vi "sc5511a_soft_front_panel.vi"() -> ()   [LabVIEW 2010]
panel:
  out "message":string="List/Sweep Mode Disabled"
  out "On":bool
  in  "stop":bool
  in  "Tab Control":T1(tab)
  in  "Phase":sgl min=-720 max=720 step=0.1 format="%.1f"
  in  "Spur Suppression":u8(ring) items=["Enabled", "Disabled"]
  in  "AutoLevel":u8(ring) items=["Enable", "Disable"]
  in  "Loop Gain":u8(ring) items=["Normal", "Low"]
  in  "Ref. Out Freq":u8(ring) items=["10 MHz", "100 MHz"]
  in  "Ref. Clock Source":u8(ring) items=["Internal 10 MHz", "Lock to External"]
  in  "RF1 Standby":bool
  in  "Lock Mode":u8(ring) items=["Harmonic Lock", "Frac-N Lock"]
  in  "ALC MODE":u8(ring) items=["Closed", "Opened"]
  in  "Power":sgl=30.0 min=-40 max=30 format="%.2f"
  in  "Interval (s)":u16=5
  in  "GetStatus":bool
  in  "Trigger":bool
  out "Device Status":T2={"Synth Mode"=1, "RF Out"=0, "Auto Level"=0, "ALC Mode"=1, "Standby"=1, "Rf RF Mode"=0, "List Mode State"=0, "RF2 Standby"=0, "Ref Lock Enable"=1, "Ext Ref Detected"=1, "Ref out mode"=1, "Main PLL"=1, "Crs PLL"=1, "Fine PLL"=1, "device accessed"=0, "Over Temp"=0, "MainLED"=FALSE, "CrsLED"=FALSE, "FineLED"=FALSE} {"Over Temp" items=["Normal", "Over Temp"]; "Ref out mode" items=["10 MHz", "100 MHz"]; "device accessed" items=["NO", "YES"]; "RF2 Standby" items=["Disabled", "Enabled"]; "Standby" items=["Disable", "Enabled"]; "Auto Level" items=["Enable", "Disable"]; "Ext Ref Detected" items=["Not Detected", "Detected"]; "Ref Lock Enable" items=["Disabled", "Enabled"]; "RF Out" items=["Disabled", "Enabled"]; "ALC Mode" items=["Closed", "Opened"]; "Rf RF Mode" items=["Single Tone", "List/Sweep"]; "Synth Mode" items=["Harmonic", "FracN"]; "List Mode State" items=["Not Triggered", "Triggered"]; "Main PLL" items=["NOT Locked", "Locked"]; "Crs PLL" items=["NOT Locked", "Locked"]; "Fine PLL" items=["NOT Locked", "Locked"]}
  in  "RF Frequency":dbl=2005000000.0 min=80000000.0 max=21000000000.0 step=1.0 format="%.9p"
  in  "RF Mode":u8(ring) items=["Single Tone", "List/Sweep"]
  in  "RF Enable":bool
  in  "RF2 Freq":sgl=6000.0 min=25 max=6000 step=25
  in  "RF2 Standby":bool
  in  "Set As Default":bool
  in  "Dwell Period (ms)":dbl=10.0 min=0.0 step=0.5 format="%.1f"
  in  "Sweep/List Cycles":u32
  in  "Sweep Freq Parameter":T3={"Start Frequency"=10040000000, "Stop Frequency"=10050000000, "Step Frequency"=100000} {"Step Frequency" max=6500000000 format="%.9p"; "Stop Frequency" max=21000000000 format="%.9p"; "Start Frequency" format="%.9p"}
  in  "List Mode Config":T4={"Sweep / List"=1, "Direction"=0, "Shape"=1, "Trigger Source"=1, "HW Trigger Mode"=0, "Return to Start"=0, "Trigger Out State"=1, "Trigger Out Behavior"=0} {"Trigger Out Behavior" items=["Trigger On Step", "Trigger On Cycle"]; "Trigger Out State" items=["Trigger Out Disable", "Trigger Out Enable"]; "Return to Start" items=["Stop at End", "Return to Start"]; "HW Trigger Mode" items=["Start/Stop", "Step"]; "Trigger Source" items=["Software", "Hardware"]; "Shape" items=["Sawtooth", "Triangle"]; "Direction" items=["Low to High", "High to Low"]; "Sweep / List" items=["List", "Sweep (start/stop/step)"]}
  in  "Load Config":bool
  in  "Save Buffer to EEPROM":bool
  in  "Read EEPROM to Buffer":bool
  in  "Download to Buffer":bool
  in  "Read From File":bool
  in  "Frequency List (2048 max)":u64[](array[numeric]) format="%.9p"
  out "message 2":string
  out "List Points":u32
  in  "SelfCal":bool
  out "Temperature":sgl=40.0 min=-30 max=120 format="%.1f"
  out "Device Info":T5={"Product SN"=268435879, "Hardware Rev"=2.0, "Firmware Rev"=2.0, "Manuf Date"={"Year"=14, "Month"=9, "Day"=10, "Hour"=10}} {"Firmware Rev" format="%.2g"; "Hardware Rev" format="%.2g"; "Product SN" format="%.0x"}
  out "error out":errorcluster
  # "(Deg)"
  # "MHz"
  # "Program will stop and the device will \nreinitialize after self calibration"
  # "DegC"
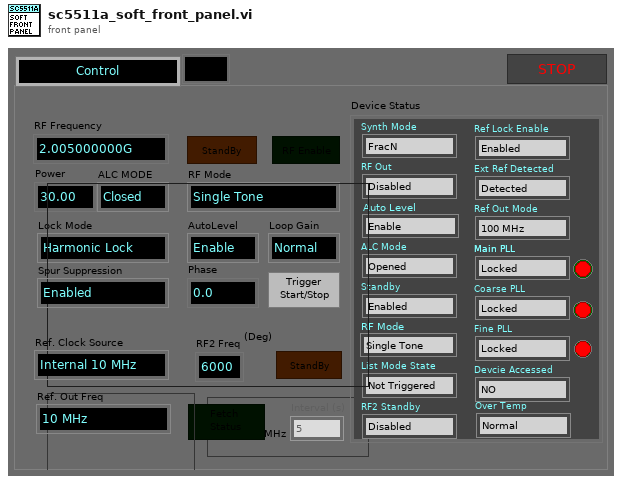
[diagram p1: front panel]
types:
  T1 = enum32{"Control", "Config Sweep/List", "List Entry", "Device Info"}
  T2 = cluster{"Synth Mode":u16, "RF Out":u16, "Auto Level":u16, "ALC Mode":u16, "Standby":u16, "Rf RF Mode":u16, "List Mode State":u16, "RF2 Standby":u16, "Ref Lock Enable":u16, "Ext Ref Detected":u16, "Ref out mode":u16, "Main PLL":u8, "Crs PLL":u8, "Fine PLL":u8, "device accessed":u16, "Over Temp":u16, "MainLED":bool, "CrsLED":bool, "FineLED":bool}
  T3 = cluster{"Start Frequency":u64, "Stop Frequency":u64, "Step Frequency":u64}
  T4 = cluster{"Sweep / List":u8, "Direction":u8, "Shape":u8, "Trigger Source":u8, "HW Trigger Mode":u8, "Return to Start":u8, "Trigger Out State":u8, "Trigger Out Behavior":u8}
  T5 = cluster{"Product SN":u32, "Hardware Rev":sgl, "Firmware Rev":sgl, "Manuf Date":cluster{"Year":u8, "Month":u8, "Day":u8, "Hour":u8}}
  T6 = cluster{"Product SN":u32, "Hardware Rev":sgl, "Firmware Rev":sgl, "Manuf Date":cluster{"Year":u32, "Month":u32, "Day":u32, "hour":u32}}
  T7 = enum32{"Control", "Config Sweep/List", "List Entry"}
  T8 = enum8{"Enabled", "Disabled", "Disabled and Grayed Out"}
  T9 = cluster{"Synth Mode":u16, "RF Out":u16, "Auto Power":u16, "ALC Mode":u16, "Standby":u16, "Rf RF Mode":u16, "List Mode State":u16, "RF2 Standby":u16, "Ref Lock Enable":u16, "Ext Ref Detected":u16, "Ref out mode":u16, "Main PLL":u8, "Crs PLL":u8, "Fine PLL":u8, "device accessed":u16, "Over Temp":u16, "MainLED":bool, "CrsLED":bool, "FineLED":bool}
  T10 = cluster{"Product SN":u32, "Hardware Rev":sgl, "Firmware Rev":sgl, "Manufacture Date":cluster{"Year":u8, "Month":u8, "Day":u8, "hour":u8}}
  T11 = cluster{"List Mode Config":cluster{"List/SSS":u8, "Direction":u8, "Shape":u8, "Trigger Source":u8, "HW Trigger Mode":u8, "Return to Start":u8, "Trigger Out State":u8, "Trigger Out Behavior":u8}, "Operate Status":cluster{"Lock Mode":u8, "Loop Gain":u8, "Device Accessed":u8, "RF2 Standby":u8, "RF1 Standby":u8, "AutoPwrLevel":u8, "AlcMode":u8, "RFOutState":u8, "Ref Lock Enable":u8, "ExtRefDetected":u8, "RefOutSelect":u8, "ListRuning":u8, "RF Mode":u8, "OverTempStatus":u8, "Harmonic SS":u8}, "PLL Status":cluster{"Sum PLL":u8, "Crs PLL":u8, "Fine PLL":u8, "Crs Ref PLL":u8, "Crs assist PLL":u8, "Ref Clk PLL":u8, "Clk 10 PLL":u8, "Lo2 PLL":u8}}
  T12 = cluster{"RF1 Freq":u64, "Sweep Start Freq":u64, "Sweep Stop Freq":u64, "Sweep Step Freq":u64, "Sweep dwell time (.5ms)":u32, "Sweep Cycles":u32, "List Buffer Points":u32, "RF1 Level (dBm)":sgl, "RF2 freq":u16}
  T13 = cluster{"List/SSS":u8, "Direction":u8, "Shape":u8, "Trigger Source":u8, "HW Trigger Mode":u8, "Return to Start":u8, "Trigger Out State":u8, "Trigger Out Behavior":u8}
  T14 = cluster{"Sweep Start Freq":u64, "Sweep Stop Freq":u64, "Sweep Step Freq":u64}
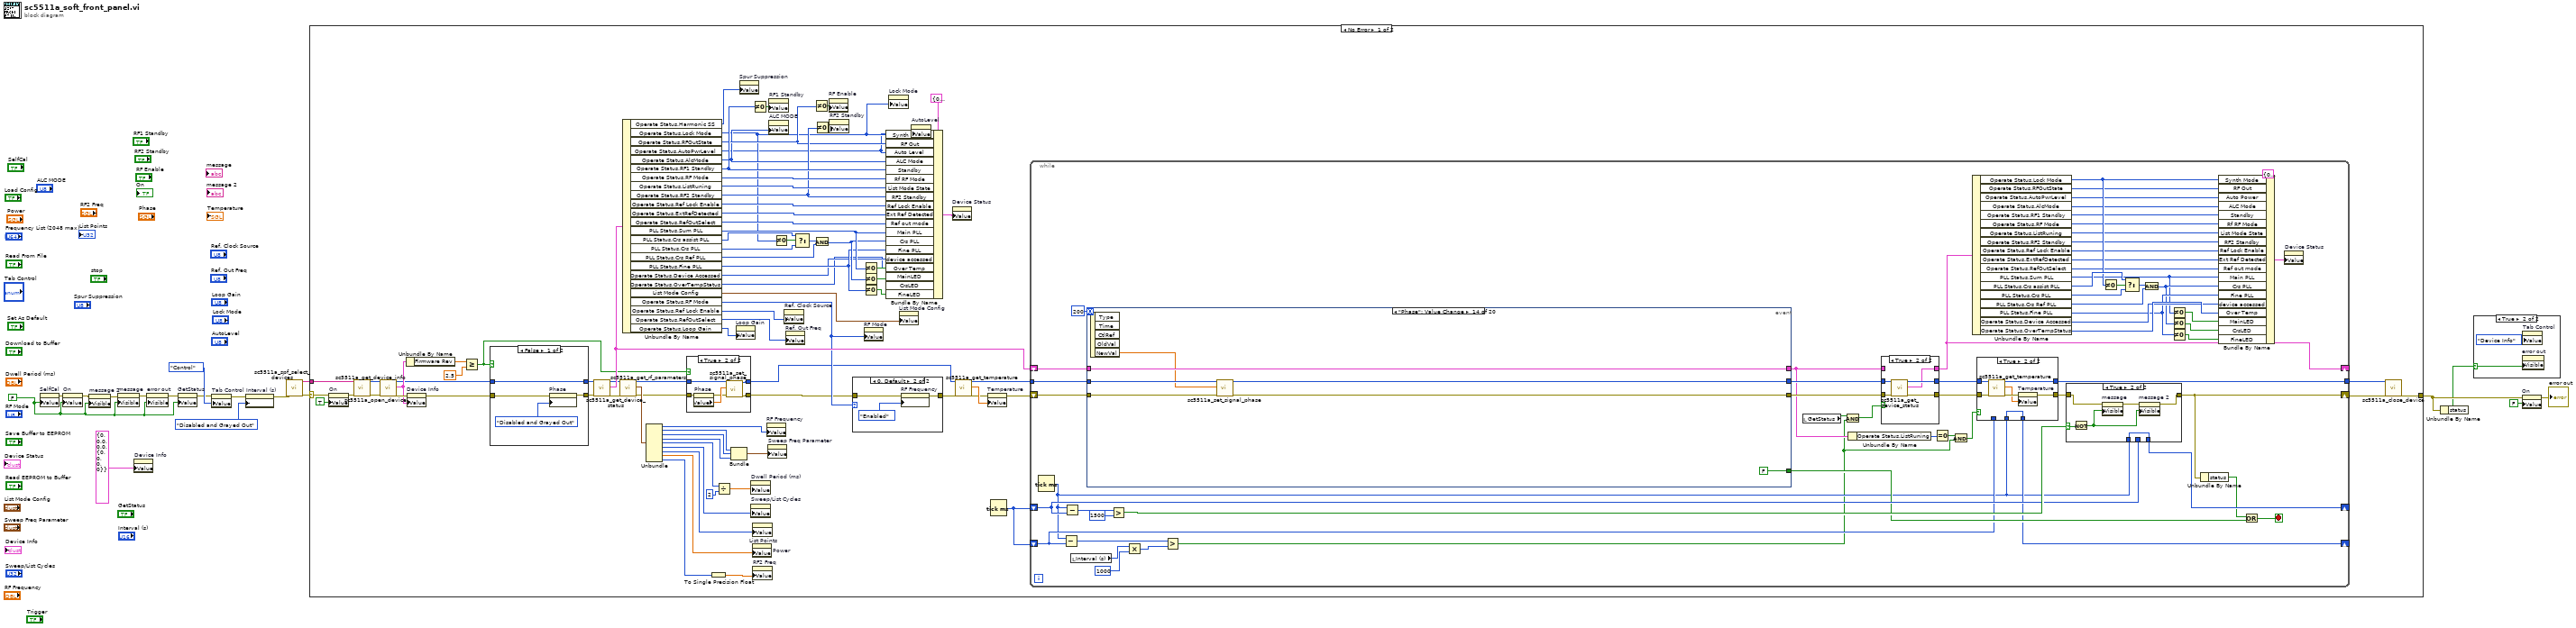
[diagram p0: block diagram]
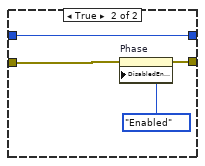
[diagram p4: hidden frame]
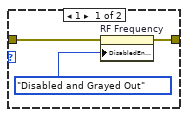
[diagram p5: hidden frame]
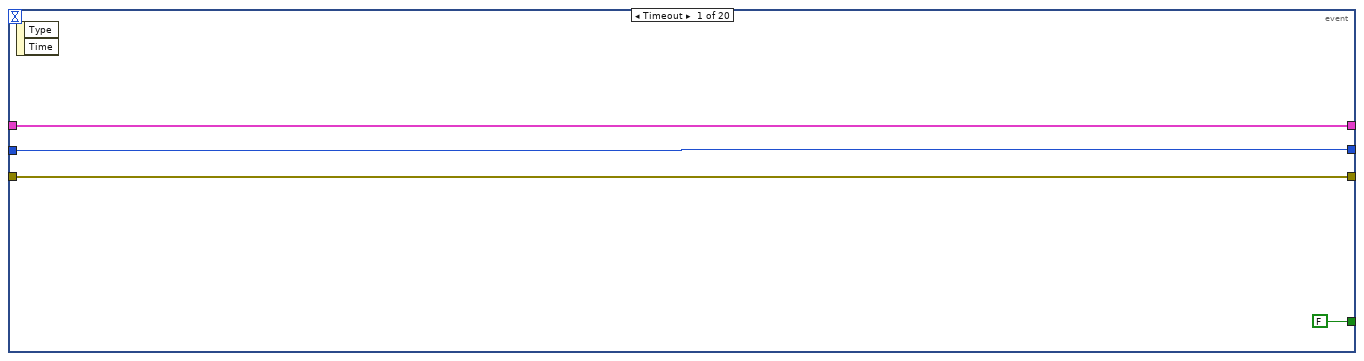
[diagram p9: hidden frame]
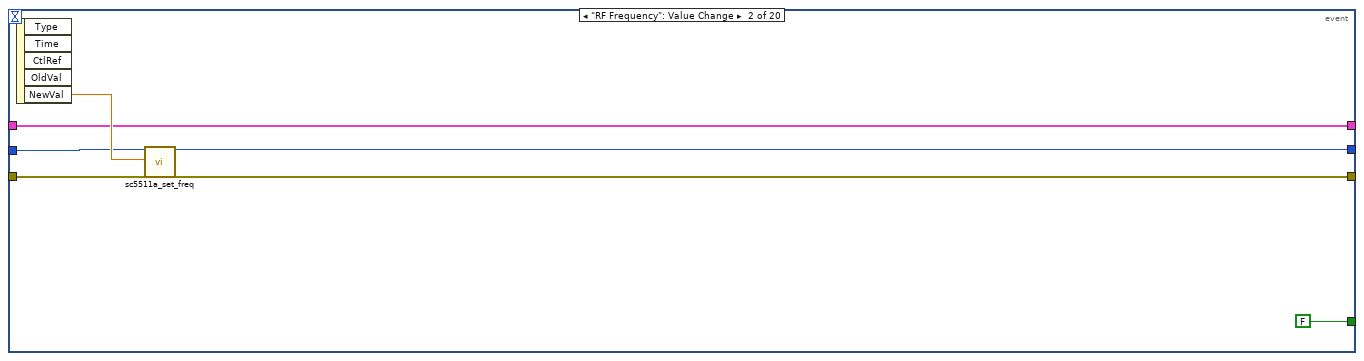
[diagram p10: hidden frame]
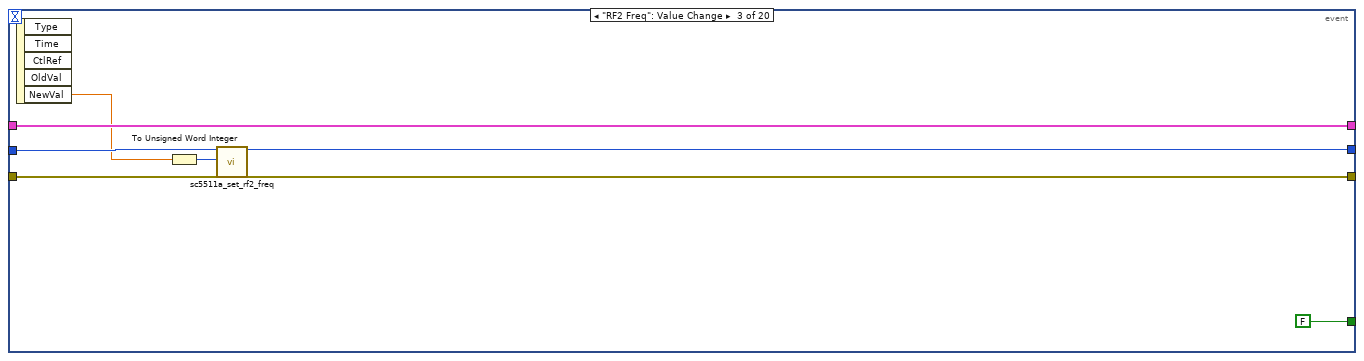
[diagram p11: hidden frame]
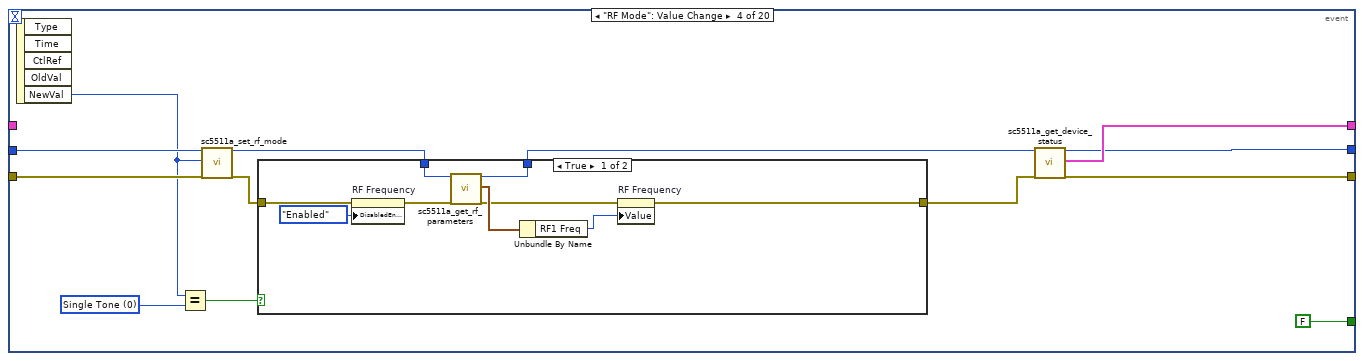
[diagram p12: hidden frame]
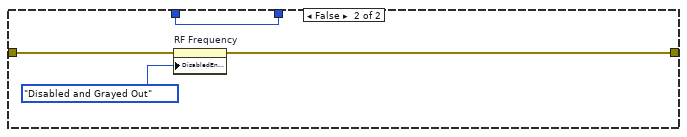
[diagram p13: hidden frame]
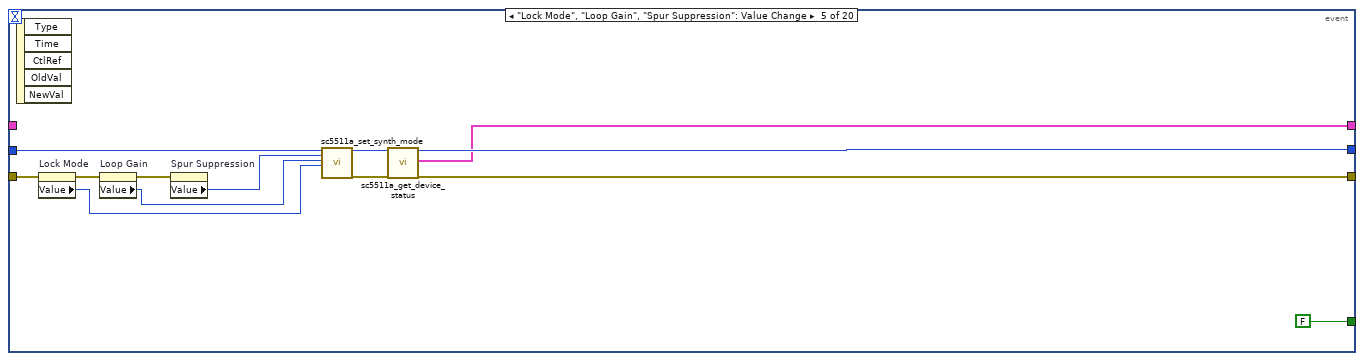
[diagram p14: hidden frame]
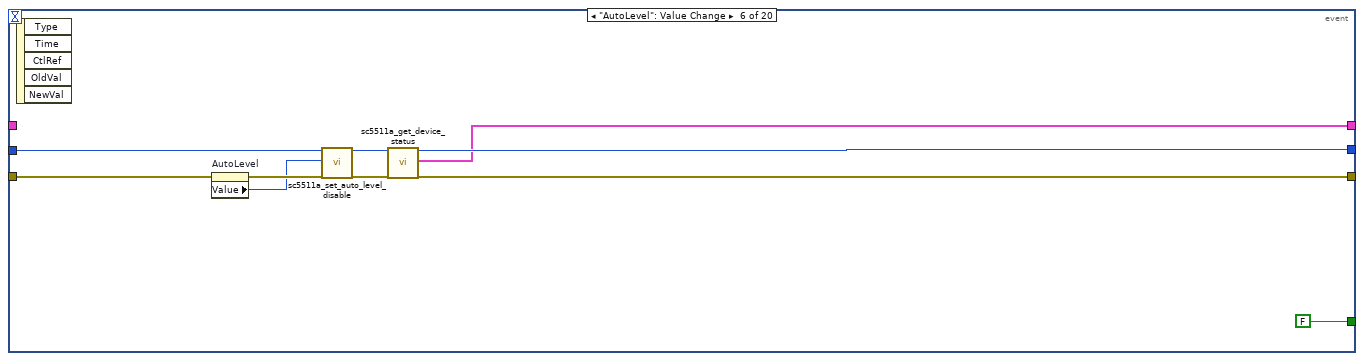
[diagram p15: hidden frame]
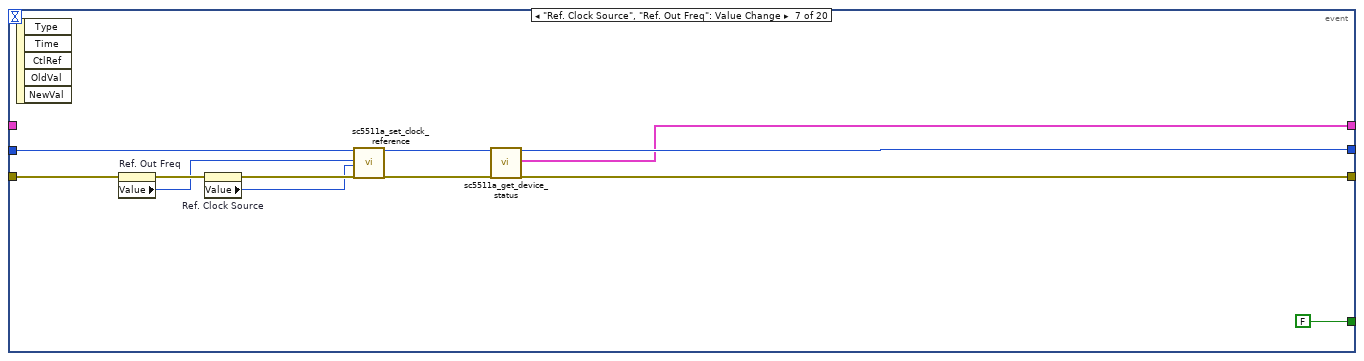
[diagram p16: hidden frame]
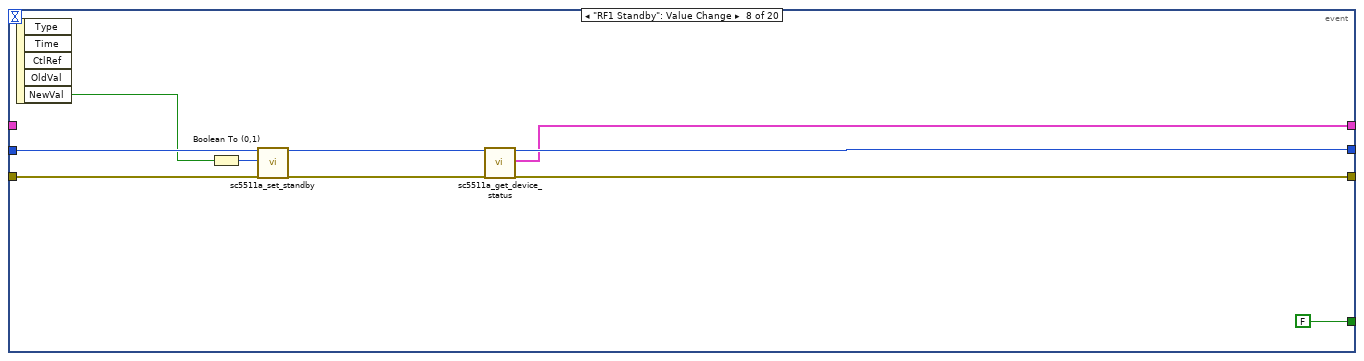
[diagram p17: hidden frame]
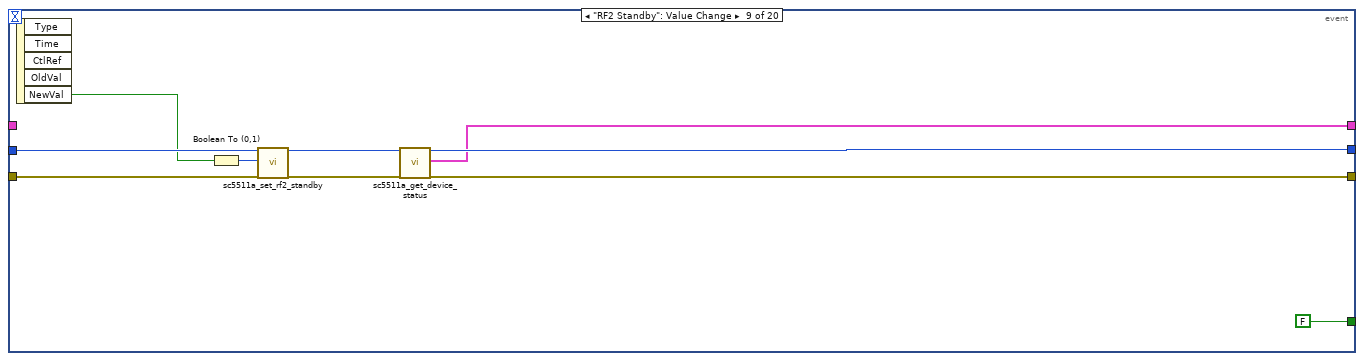
[diagram p18: hidden frame]
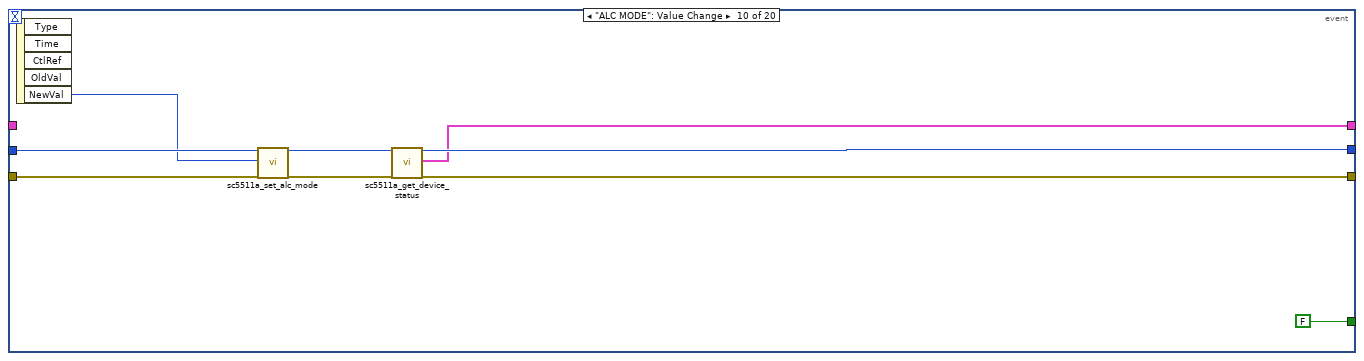
[diagram p19: hidden frame]
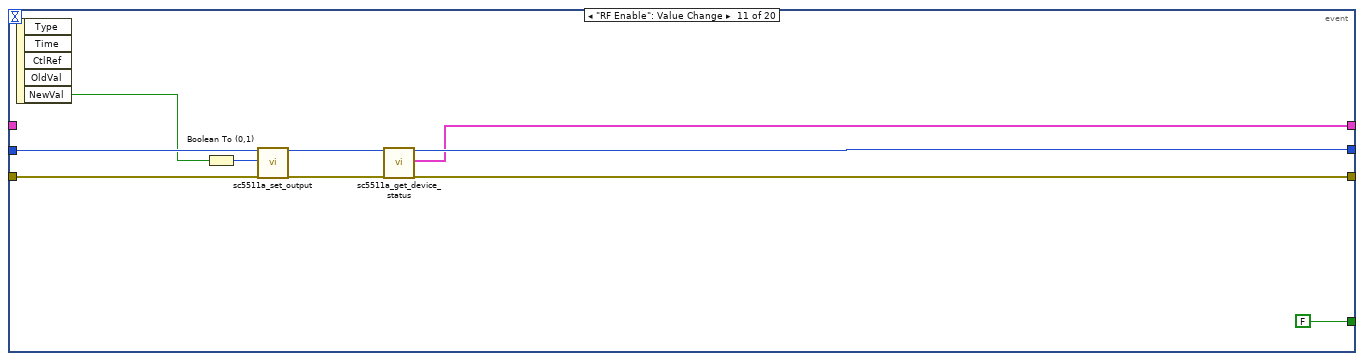
[diagram p20: hidden frame]
diagram:
  w1 = FALSE ("Visible")
  n1 = property on="SelfCal" class="Bool (strict)"("Value"=w1) -> (error out=w2:errorcluster)  [unwired: 2 in, 1 out]
  n2 = property on="On" class="Bool (strict)"(error in=w2, "Value"=w1) -> (error out=w4:errorcluster)  [unwired: 1 in, 1 out]
  n3 = property on="message 2" class="Str"(error in=w4, "Visible"=w1) -> (error out=w18:errorcluster)  [unwired: 1 in, 1 out]
  n4 = property on="message" class="Str"(error in=w18, "Visible"=w1) -> (error out=w17:errorcluster)  [unwired: 1 in, 1 out]
  n5 = property on="Device Info" class="Clust (strict)"("Value"=T6 {"Product SN"=0, "Hardware Rev"=0.0, "Firmware Rev"=0.0, "Manuf Date"={"Year"=0, "Month"=0, "Day"=0, "hour"=0}} ("Device Info")) -> ()  [unwired: 2 in, 2 out]
  n6 = property on="error out" class="Clust (strict)"(error in=w17, "Visible"=w1) -> (error out=w15:errorcluster)  [unwired: 1 in, 1 out]
  n7 = property on="GetStatus" class="Bool (strict)"(error in=w15, "Value"=w1) -> (error out=w10:errorcluster)  [unwired: 1 in, 1 out]
  n8 = property on="Tab Control" class="TabCtl (strict)"(error in=w10, "Value"=T7."Control" ("Tab Control")) -> (error out=w11:errorcluster)  [unwired: 1 in, 1 out]
  n9 = property on="Interval (s)" class="DigNum (strict)"(error in=w11, "DisabledEnum"=T8."Disabled and Grayed Out" ("Disabled")) -> (error out=w14:errorcluster)  [unwired: 1 in, 1 out]
  n10 = call "sc5511a_spf_select_devices.vi"("error in (no error)"=w14) -> ("Selected Resource"=w8:string, "error out"=w16:errorcluster)  [unwired: 17 in]
  n11 = case shown="No Error" w16 {
    selector: w16 -> [w84 w578]
    tunnel: [w96 w578] -> w7
    tunnel: w8 -> [w83 _]
    frame No Error {
      n12 = property on="On" class="Bool (strict)"(error in=w84, "Value"=TRUE ("Visible")) -> (error out=w85:errorcluster)  [unwired: 1 in, 1 out]
      n13 = call "sc5511a_open_device.vi"("Device SN String"=w83, "error in (no error)"=w85) -> ("deviceHandle"=w87:u32, "error out"=w88:errorcluster)  [unwired: 16 in]
      n14 = call "sc5511a_get_device_info.vi"("deviceHandle"=w87, "error in"=w88) -> ("deviceHandle"=w22:u32, "Device Info"=w27:T10, "error out"=w93:errorcluster)  [unwired: 15 in]
      n15 = Unbundle By Name(w27) -> ("Firmware Rev"=w26:sgl)
      n16 = property on="Device Info" class="Clust (strict)"(error in=w93, "Value"=w27) -> (error out=w23:errorcluster)  [unwired: 1 in, 1 out]
      n17 = Greater Or Equal?(x=w26, y=sgl 2.5) -> (x >= y?=w19:bool)
      n18 = case shown="False" w19 {
        tunnel: [w108 w113] -> w24
        tunnel: w23 -> [w109 w112]
        tunnel: w22 -> [w110 w114]
        tunnel: [w110 w114] -> w21
        frame False {
          n19 = property on="Phase" class="DigNum (strict)"(error in=w109, "DisabledEnum"=T8."Disabled and Grayed Out" ("Disabled")) -> (error out=w108:errorcluster)  [unwired: 1 in, 1 out]
        }
        frame True {
          n20 = property on="Phase" class="DigNum (strict)"(error in=w112, "DisabledEnum"=T8."Enabled" ("Disabled")) -> (error out=w113:errorcluster)  [unwired: 1 in, 1 out]
        }
      }
      n21 = call "sc5511a_get_device_status.vi"("deviceHandle"=w21, "error in"=w24) -> ("deviceHandle"=w80:u32, "Device Status"=w94:T11, "error out"=w81:errorcluster)  [unwired: 15 in]
      n22 = call "sc5511a_get_rf_parameters.vi"("deviceHandle"=w80, "error in"=w81) -> ("deviceHandle"=w29:u32, "RF Params"=w79:T12, "error out"=w20:errorcluster)  [unwired: 15 in]
      n23 = Unbundle By Name(w94) -> ("Operate Status.Harmonic SS"=w31:u8, "Operate Status.Lock Mode"=w35:u8, "Operate Status.RFOutState"=w43:u8, "Operate Status.AutoPwrLevel"=w32:u8, "Operate Status.AlcMode"=w42:u8, "Operate Status.RF1 Standby"=w48:u8, "Operate Status.RF Mode"=w65:u8, "Operate Status.ListRuning"=w64:u8, "Operate Status.RF2 Standby"=w44:u8, "Operate Status.Ref Lock Enable"=w63:u8, "Operate Status.ExtRefDetected"=w62:u8, "Operate Status.RefOutSelect"=w61:u8, "PLL Status.Sum PLL"=w60:u8, "PLL Status.Crs assist PLL"=w56:u8, "PLL Status.Crs PLL"=w55:u8, "PLL Status.Crs Ref PLL"=w57:u8, "PLL Status.Fine PLL"=w53:u8, "Operate Status.Device Accessed"=w52:u8, "Operate Status.OverTempStatus"=w51:u8, "List Mode Config"=w95:T13, "Operate Status.RF Mode"=w86:u8, "Operate Status.Ref Lock Enable"=w50:u8, "Operate Status.RefOutSelect"=w49:u8, "Operate Status.Loop Gain"=w36:u8)
      n24 = Unbundle(w79) -> ("RF1 Freq"=w78:u64, "Sweep Start Freq"=w76:u64, "Sweep Stop Freq"=w75:u64, "Sweep Step Freq"=w74:u64, "Sweep dwell time (.5ms)"=w71:u32, "Sweep Cycles"=w73:u32, "List Buffer Points"=w69:u32, "RF1 Level (dBm)"=w68:sgl, "RF2 freq"=w66:u16)
      n25 = case shown="True" w19 {
        tunnel: [w99 w106] -> w30
        tunnel: w29 -> [w100 w105]
        tunnel: [w100 w104] -> w28
        tunnel: w20 -> [w99 w102]
        frame False {
        }
        frame True {
          n26 = property on="Phase" class="DigNum (strict)"(error in=w102) -> (error out=w101:errorcluster, "Value"=w103:sgl)  [unwired: 1 in, 1 out]
          n27 = call "sc5511a_set_signal_phase.vi"("deviceHandle"=w105, "Phase (deg)"=w103, "error in"=w101) -> ("deviceHandle"=w104:u32, "error out"=w106:errorcluster)  [unwired: 15 in]
        }
      }
      n28 = To Single Precision Float(number=w66) -> (single precision float=w67:sgl)
      n29 = Divide(x=w71, y=u32 2) -> (x/y=w72:dbl)
      n30 = Bundle("Sweep Start Freq"=w76, "Sweep Stop Freq"=w75, "Sweep Step Freq"=w74) -> (w77:T14)  [unwired: 1 in]
      n31 = property on="Loop Gain" class="Ring (strict)"("Value"=w36) -> ()  [unwired: 2 in, 2 out]
      n32 = property on="Spur Suppression" class="Ring (strict)"("Value"=w31) -> ()  [unwired: 2 in, 2 out]
      n33 = property on="Dwell Period (ms)" class="DigNum (strict)"("Value"=w72) -> ()  [unwired: 2 in, 2 out]
      n34 = property on="Sweep/List Cycles" class="DigNum (strict)"("Value"=w73) -> ()  [unwired: 2 in, 2 out]
      n35 = Not Equal To 0?(x=w48) -> (x != 0?=w47:bool)
      n36 = property on="Power" class="DigNum (strict)"("Value"=w68) -> ()  [unwired: 2 in, 2 out]
      n37 = property on="List Points" class="DigNum (strict)"("Value"=w69) -> ()  [unwired: 2 in, 2 out]
      n38 = property on="RF2 Freq" class="DigNum (strict)"("Value"=w67) -> ()  [unwired: 2 in, 2 out]
      n39 = property on="RF Frequency" class="DigNum (strict)"("Value"=w78) -> ()  [unwired: 2 in, 2 out]
      n40 = property on="Sweep Freq Parameter" class="Clust (strict)"("Value"=w77) -> ()  [unwired: 2 in, 2 out]
      n41 = property on="RF1 Standby" class="Bool (strict)"("Value"=w47) -> ()  [unwired: 2 in, 2 out]
      n42 = property on="ALC MODE" class="Ring (strict)"("Value"=w42) -> ()  [unwired: 2 in, 2 out]
      n43 = Not Equal To 0?(x=w35) -> (x != 0?=w59:bool)
      n44 = property on="Ref. Clock Source" class="Ring (strict)"("Value"=w50) -> ()  [unwired: 2 in, 2 out]
      n45 = property on="Ref. Out Freq" class="Ring (strict)"("Value"=w49) -> ()  [unwired: 2 in, 2 out]
      n46 = Select(t=w56, s=w59, f=w55) -> (s? t:f=w58:u8)
      n47 = Not Equal To 0?(x=w43) -> (x != 0?=w46:bool)
      n48 = Not Equal To 0?(x=w44) -> (x != 0?=w45:bool)
      n49 = And(x=w58, y=w57) -> (x .and. y?=w54:u8)
      n50 = property on="RF Enable" class="Bool (strict)"("Value"=w46) -> ()  [unwired: 2 in, 2 out]
      n51 = property on="RF2 Standby" class="Bool (strict)"("Value"=w45) -> ()  [unwired: 2 in, 2 out]
      n52 = case shown="0, Default" w86 {
        tunnel: w30 -> [w116 w119]
        tunnel: [w115 w118] -> w40
        frame 1 {
          n53 = property on="RF Frequency" class="DigNum (strict)"(error in=w116, "DisabledEnum"=T8."Disabled and Grayed Out" ("Disabled")) -> (error out=w115:errorcluster)  [unwired: 1 in, 1 out]
        }
        frame 0, Default {
          n54 = property on="RF Frequency" class="DigNum (strict)"(error in=w119, "DisabledEnum"=T8."Enabled" ("Disabled")) -> (error out=w118:errorcluster)  [unwired: 1 in, 1 out]
        }
      }
      n55 = Not Equal To 0?(x=w60) -> (x != 0?=w91:bool)
      n56 = Not Equal To 0?(x=w54) -> (x != 0?=w90:bool)
      n57 = Not Equal To 0?(x=w53) -> (x != 0?=w89:bool)
      n58 = property on="RF Mode" class="Ring (strict)"("Value"=w86) -> ()  [unwired: 2 in, 2 out]
      n59 = Bundle By Name(cluster=T2 {"Synth Mode"=0, "RF Out"=1, "Auto Level"=1, "ALC Mode"=0, "Standby"=0, "Rf RF Mode"=0, "List Mode State"=0, "RF2 Standby"=1, "Ref Lock Enable"=0, "Ext Ref Detected"=0, "Ref out mode"=0, "Main PLL"=1, "Crs PLL"=1, "Fine PLL"=1, "device accessed"=1, "Over Temp"=0, "MainLED"=TRUE, "CrsLED"=TRUE, "FineLED"=TRUE} ("Device Status"), "Synth Mode"=w35, "RF Out"=w43, "Auto Level"=w32, "ALC Mode"=w42, "Standby"=w48, "Rf RF Mode"=w65, "List Mode State"=w64, "RF2 Standby"=w44, "Ref Lock Enable"=w63, "Ext Ref Detected"=w62, "Ref out mode"=w61, "Main PLL"=w60, "Crs PLL"=w54, "Fine PLL"=w53, "device accessed"=w52, "Over Temp"=w51, "MainLED"=w91, "CrsLED"=w90, "FineLED"=w89) -> (w34:T2)
      n60 = property on="Lock Mode" class="Ring (strict)"("Value"=w35) -> ()  [unwired: 2 in, 2 out]
      n61 = property on="List Mode Config" class="Clust (strict)"("Value"=w95) -> ()  [unwired: 2 in, 2 out]
      n62 = property on="AutoLevel" class="Ring (strict)"("Value"=w32) -> ()  [unwired: 2 in, 2 out]
      n63 = property on="Device Status" class="Clust (strict)"("Value"=w34) -> ()  [unwired: 2 in, 2 out]
      n64 = call "sc5511a_get_temperature.vi"("deviceHandle"=w28, "error in"=w40) -> ("deviceHandle"=w41:u32, "temperature"=w39:sgl, "error out"=w37:errorcluster)  [unwired: 15 in]
      n65 = property on="Temperature" class="DigNum (strict)"(error in=w37, "Value"=w39) -> (error out=w38:errorcluster)  [unwired: 1 in, 1 out]
      n66 = Tick Count (ms)() -> (millisecond timer value=w92:u32)
      n67 = while {
        shift-right: [w162] -> w98
        shift-left: w38 -> [w180]
        tunnel: w41 -> [w179]
        tunnel: [w129] -> w97
        shift-right: [w137] -> _
        shift-left: w94 -> [w176]
        shift-right: [w166] -> _
        shift-left: w92 -> [w165]
        shift-right: [w132] -> _
        shift-left: w92 -> [w133]
        stop <- w161 stop-if-true
        n68 = Tick Count (ms)() -> (millisecond timer value=w131:u32)
        n69 = Subtract(x=w131, y=w133) -> (x-y=w170:u32)
        n70 = Subtract(x=w131, y=w165) -> (x-y=w175:u32)
        n71 = local read "Interval (s)"() -> (w171:u16)
        n72 = event shown="[13] \"Phase\": Value Change" {
          selector: _ -> [_ _ _ _ _ _ _ _ _ _ _ _ _ _ _ _ _ _ _ _]
          dyn-events: _ -> [_ _ _ _ _ _ _ _ _ _ _ _ _ _ _ _ _ _ _ _]
          timeout: 200 -> [_ _ _ _ _ _ _ _ _ _ _ _ _ _ _ _ _ _ _ _]
          tunnel: w179 -> [w209 w216 w225 w236 w263 w273 w285 w294 w304 w313 w323 w329 w346 w354 w358 w379 w390 w462 w477 w524]
          tunnel: w180 -> [w210 w215 w224 w237 w257 w265 w284 w295 w305 w314 w324 w328 w347 w352 w363 w376 w391 w461 w478 w525]
          tunnel: [w209 w213 w222 w228 w260 w270 w276 w289 w300 w309 w318 w332 w345 w350 w359 w379 w383 w438 w476 w519] -> w178
          tunnel: [w210 w214 w223 w229 w262 w272 w279 w290 w301 w311 w320 w333 w344 w351 w360 w377 w385 w436 w475 w520] -> w177
          tunnel: w176 -> [w208 w212 w221 _ _ _ _ _ _ _ _ _ w349 w356 _ w380 w386 w434 w470 w517]
          tunnel: [w208 w212 w221 w231 w258 w268 w275 w287 w297 w307 w316 w331 w349 w356 w357 w380 w381 w434 w470 w517] -> w126
          tunnel: [FALSE ("NewVal") FALSE FALSE FALSE FALSE FALSE FALSE FALSE FALSE FALSE FALSE w330 FALSE FALSE FALSE TRUE ("NewVal") FALSE ("NewVal") FALSE ("NewVal") FALSE ("NewVal") FALSE ("NewVal")] -> w164
          event Timeout {
            n73 = event-data() -> ()  [unwired: 1 in, 2 out]
          }
          event "RF Frequency": Value Change {
            n74 = event-data() -> ("NewVal"=w217:dbl)  [unwired: 1 in, 4 out]
            n75 = call "sc5511a_set_freq.vi"("deviceHandle"=w216, "RF1 frequency"=w217, "error in"=w215) -> ("deviceHandle"=w213:u32, "error out"=w214:errorcluster)  [unwired: 15 in]
          }
          event "RF2 Freq": Value Change {
            n76 = event-data() -> ("NewVal"=w218:sgl)  [unwired: 1 in, 4 out]
            n77 = To Unsigned Word Integer(number=w218) -> (unsigned 16bit integer=w219:u16)
            n78 = call "sc5511a_set_rf2_freq.vi"("deviceHandle"=w225, "RF1 frequency (MHz)"=w219, "error in"=w224) -> ("deviceHandle"=w222:u32, "error out"=w223:errorcluster)  [unwired: 15 in]
          }
          event "RF Mode": Value Change {
            w234 = u8 0 items=["Single Tone", "List/Sweep"] ("RF Mode")
            n79 = event-data() -> ("NewVal"=w233:u8)  [unwired: 1 in, 4 out]
            n80 = Equal?(x=w233, y=w234) -> (x = y?=w232:bool)
            n81 = call "sc5511a_set_rf_mode.vi"("deviceHandle"=w236, "RF Mode"=w233, "error in"=w237) -> ("deviceHandle"=w227:u32, "error out"=w235:errorcluster)  [unwired: 15 in]
            n82 = case shown="True" w232 {
              tunnel: w235 -> [w247 w251]
              tunnel: [w239 w250] -> w230
              tunnel: w227 -> [w244 w248]
              tunnel: [w243 w248] -> w226
              frame True {
                n83 = property on="RF Frequency" class="DigNum (strict)"(error in=w247, "DisabledEnum"=T8."Enabled" ("Disabled")) -> (error out=w245:errorcluster)  [unwired: 1 in, 1 out]
                n84 = call "sc5511a_get_rf_parameters.vi"("deviceHandle"=w244, "error in"=w245) -> ("deviceHandle"=w243:u32, "RF Params"=w242:T12, "error out"=w240:errorcluster)  [unwired: 15 in]
                n85 = Unbundle By Name(w242) -> ("RF1 Freq"=w241:u64)
                n86 = property on="RF Frequency" class="DigNum (strict)"(error in=w240, "Value"=w241) -> (error out=w239:errorcluster)  [unwired: 1 in, 1 out]
              }
              frame False {
                n87 = property on="RF Frequency" class="DigNum (strict)"(error in=w251, "DisabledEnum"=T8."Disabled and Grayed Out" ("Disabled")) -> (error out=w250:errorcluster)  [unwired: 1 in, 1 out]
              }
            }
            n88 = call "sc5511a_get_device_status.vi"("deviceHandle"=w226, "error in"=w230) -> ("deviceHandle"=w228:u32, "Device Status"=w231:T11, "error out"=w229:errorcluster)  [unwired: 15 in]
          }
          event "Lock Mode", "Loop Gain", "Spur Suppression": Value Change {
            n89 = event-data() -> ()  [unwired: 1 in, 5 out]
            n90 = property on="Lock Mode" class="Ring (strict)"(error in=w257) -> (error out=w256:errorcluster, "Value"=w254:u8)  [unwired: 1 in, 1 out]
            n91 = property on="Loop Gain" class="Ring (strict)"(error in=w256) -> (error out=w253:errorcluster, "Value"=w255:u8)  [unwired: 1 in, 1 out]
            n92 = property on="Spur Suppression" class="Ring (strict)"(error in=w253) -> ("Value"=w252:u8)  [unwired: 1 in, 2 out]
            n93 = call "sc5511a_set_synth_mode.vi"("deviceHandle"=w263, "Harmonic Spur Suppression"=w252, "loop gain"=w255, "lock mode"=w254) -> ("deviceHandle"=w259:u32, "error out"=w261:errorcluster)  [unwired: 14 in]
            n94 = call "sc5511a_get_device_status.vi"("deviceHandle"=w259, "error in"=w261) -> ("deviceHandle"=w260:u32, "Device Status"=w258:T11, "error out"=w262:errorcluster)  [unwired: 15 in]
          }
          event "AutoLevel": Value Change {
            n95 = event-data() -> ()  [unwired: 1 in, 5 out]
            n96 = property on="AutoLevel" class="Ring (strict)"(error in=w265) -> (error out=w267:errorcluster, "Value"=w266:u8)  [unwired: 1 in, 1 out]
            n97 = call "sc5511a_set_auto_level_disable.vi"("deviceHandle"=w273, "auto leveling"=w266, "error in"=w267) -> ("deviceHandle"=w269:u32, "error out"=w271:errorcluster)  [unwired: 15 in]
            n98 = call "sc5511a_get_device_status.vi"("deviceHandle"=w269, "error in"=w271) -> ("deviceHandle"=w270:u32, "Device Status"=w268:T11, "error out"=w272:errorcluster)  [unwired: 15 in]
          }
          event "Ref. Clock Source", "Ref. Out Freq": Value Change {
            n99 = event-data() -> ()  [unwired: 1 in, 5 out]
            n100 = property on="Ref. Out Freq" class="Ring (strict)"(error in=w284) -> (error out=w283:errorcluster, "Value"=w280:u8)  [unwired: 1 in, 1 out]
            n101 = property on="Ref. Clock Source" class="Ring (strict)"(error in=w283) -> (error out=w282:errorcluster, "Value"=w281:u8)  [unwired: 1 in, 1 out]
            n102 = call "sc5511a_set_clock_reference.vi"("deviceHandle"=w285, "Ref Output"=w280, "Lock external"=w281, "error in"=w282) -> ("deviceHandle"=w277:u32, "error out"=w278:errorcluster)  [unwired: 14 in]
            n103 = call "sc5511a_get_device_status.vi"("deviceHandle"=w277, "error in"=w278) -> ("deviceHandle"=w276:u32, "Device Status"=w275:T11, "error out"=w279:errorcluster)  [unwired: 15 in]
          }
          event "RF1 Standby": Value Change {
            n104 = event-data() -> ("NewVal"=w293:bool)  [unwired: 1 in, 4 out]
            n105 = Boolean To (0,1)(Boolean=w293) -> (0, 1=w292:i16)
            n106 = call "sc5511a_set_standby.vi"("deviceHandle"=w294, "Standby"=w292, "error in"=w295) -> ("deviceHandle"=w288:u32, "error out"=w291:errorcluster)  [unwired: 15 in]
            n107 = call "sc5511a_get_device_status.vi"("deviceHandle"=w288, "error in"=w291) -> ("deviceHandle"=w289:u32, "Device Status"=w287:T11, "error out"=w290:errorcluster)  [unwired: 15 in]
          }
          event "RF2 Standby": Value Change {
            n108 = event-data() -> ("NewVal"=w303:bool)  [unwired: 1 in, 4 out]
            n109 = Boolean To (0,1)(Boolean=w303) -> (0, 1=w302:i16)
            n110 = call "sc5511a_set_rf2_standby.vi"("deviceHandle"=w304, "Standby"=w302, "error in"=w305) -> ("deviceHandle"=w299:u32, "error out"=w298:errorcluster)  [unwired: 15 in]
            n111 = call "sc5511a_get_device_status.vi"("deviceHandle"=w299, "error in"=w298) -> ("deviceHandle"=w300:u32, "Device Status"=w297:T11, "error out"=w301:errorcluster)  [unwired: 15 in]
          }
          event "ALC MODE": Value Change {
            n112 = event-data() -> ("NewVal"=w312:u8)  [unwired: 1 in, 4 out]
            n113 = call "sc5511a_set_alc_mode.vi"("deviceHandle"=w313, "alc mode"=w312, "error in"=w314) -> ("deviceHandle"=w308:u32, "error out"=w310:errorcluster)  [unwired: 15 in]
            n114 = call "sc5511a_get_device_status.vi"("deviceHandle"=w308, "error in"=w310) -> ("deviceHandle"=w309:u32, "Device Status"=w307:T11, "error out"=w311:errorcluster)  [unwired: 15 in]
          }
          event "RF Enable": Value Change {
            n115 = event-data() -> ("NewVal"=w321:bool)  [unwired: 1 in, 4 out]
            n116 = Boolean To (0,1)(Boolean=w321) -> (0, 1=w322:i16)
            n117 = call "sc5511a_set_output.vi"("deviceHandle"=w323, "RF Output"=w322, "error in"=w324) -> ("deviceHandle"=w317:u32, "error out"=w319:errorcluster)  [unwired: 15 in]
            n118 = call "sc5511a_get_device_status.vi"("deviceHandle"=w317, "error in"=w319) -> ("deviceHandle"=w318:u32, "Device Status"=w316:T11, "error out"=w320:errorcluster)  [unwired: 15 in]
          }
          event "SelfCal": Value Change {
            n119 = event-data() -> ("NewVal"=w330:bool)  [unwired: 1 in, 4 out]
            n120 = case shown="True" w330 {
              tunnel: w329 -> [w335 w342]
              tunnel: w328 -> [w334 w341]
              tunnel: [w335 w340] -> w327
              tunnel: [w334 w337] -> w326
              frame False {
              }
              frame True {
                n121 = call "sc5511a_synth_self_cal.vi"("deviceHandle"=w342, "error in"=w341) -> ("deviceHandle"=w340:u32, "error out"=w339:errorcluster)  [unwired: 16 in]
                n122 = call "Time Delay4"("error in (no error)"=w339) -> ("error out"=w338:errorcluster)  [unwired: 10 in]
                n123 = property on="SelfCal" class="Bool (strict)"(error in=w338, "Value"=FALSE ("SelfCal")) -> (error out=w337:errorcluster)  [unwired: 1 in, 1 out]
              }
            }
            n124 = call "sc5511a_get_device_status.vi"("deviceHandle"=w327, "error in"=w326) -> ("deviceHandle"=w332:u32, "Device Status"=w331:T11, "error out"=w333:errorcluster)  [unwired: 15 in]
          }
          event "Power": Value Change {
            n125 = event-data() -> ("NewVal"=w343:sgl)  [unwired: 1 in, 4 out]
            n126 = call "sc5511a_set_level.vi"("deviceHandle"=w346, "level (dBm)"=w343, "error in"=w347) -> ("deviceHandle"=w345:u32, "error out"=w344:errorcluster)  [unwired: 15 in]
          }
          event "Phase": Value Change {
            n127 = event-data() -> ("NewVal"=w353:sgl)  [unwired: 1 in, 4 out]
            n128 = call "sc5511a_set_signal_phase.vi"("deviceHandle"=w354, "Phase (deg)"=w353, "error in"=w352) -> ("deviceHandle"=w350:u32, "error out"=w351:errorcluster)  [unwired: 15 in]
          }
          event "GetStatus": Value Change {
            n129 = event-data() -> ("NewVal"=w362:bool)  [unwired: 1 in, 4 out]
            n130 = case shown="True" w362 {
              selector: w362 -> [w368 w371]
              tunnel: w363 -> [w370 w374]
              tunnel: [w365 w373] -> w361
              tunnel: [w368 w371] -> _
              frame True {
                n131 = property on="RF Frequency" class="DigNum (strict)"(error in=w370, "DisabledEnum"=T8."Enabled" ("Disabled")) -> (error out=w366:errorcluster)  [unwired: 1 in, 1 out]
                n132 = property on="Interval (s)" class="DigNum (strict)"(error in=w366, "DisabledEnum"=T8."Enabled" ("Disabled")) -> (error out=w365:errorcluster)  [unwired: 1 in, 1 out]
              }
              frame False {
                n133 = property on="Interval (s)" class="DigNum (strict)"(error in=w374, "DisabledEnum"=T8."Disabled and Grayed Out" ("Disabled")) -> (error out=w373:errorcluster)  [unwired: 1 in, 1 out]
              }
            }
            n134 = call "sc5511a_get_device_status.vi"("deviceHandle"=w358, "error in"=w361) -> ("deviceHandle"=w359:u32, "Device Status"=w357:T11, "error out"=w360:errorcluster)  [unwired: 15 in]
          }
          event "stop": Value Change {
            n135 = event-data() -> ()  [unwired: 1 in, 5 out]
            n136 = property on="stop" class="Bool (strict)"(error in=w376, "Value"=FALSE ("stop")) -> (error out=w377:errorcluster)  [unwired: 1 in, 1 out]
          }
          event "Trigger": Value Change {
            (unwired) u16 0 ("ListMode State")
            n137 = event-data() -> ()  [unwired: 1 in, 5 out]
            n138 = Unbundle By Name(w386) -> ("Operate Status.RF Mode"=w394:u8, "Operate Status.ListRuning"=w393:u8, "List Mode Config.Trigger Source"=w392:u8)
            n139 = case shown="1" w394 {
              tunnel: w393 -> [_ w406]
              tunnel: w392 -> [_ w405]
              tunnel: w391 -> [w397 w404]
              tunnel: [w396 w403] -> w388
              tunnel: w390 -> [w400 w402]
              tunnel: [w400 w401] -> w382
              frame 0, Default {
                n140 = property on="message" class="Str"(error in=w397, "Visible"=TRUE, "Value"="List/Sweep Mode Disabled" ("hwtrigSel'd")) -> (error out=w396:errorcluster)  [unwired: 1 in, 1 out]
              }
              frame 1 {
                n141 = case shown="0, Default" w406 {
                  tunnel: w405 -> [w411 _]
                  tunnel: w404 -> [w410 w423]
                  tunnel: [w409 w422] -> w403
                  tunnel: w402 -> [w408 w424]
                  tunnel: [w407 w421] -> w401
                  frame 0, Default {
                    n142 = case shown="1" w411 {
                      tunnel: [w414 w419] -> w409
                      tunnel: w410 -> [w415 w420]
                      tunnel: w408 -> [w413 w416]
                      tunnel: [w412 w416] -> w407
                      frame 0, Default {
                        n143 = call "sc5511a_list_soft_trigger.vi"("deviceHandle"=w413, "error in"=w415) -> ("deviceHandle"=w412:u32, "error out"=w414:errorcluster)  [unwired: 16 in]
                      }
                      frame 1 {
                        n144 = property on="message" class="Str"(error in=w420, "Visible"=TRUE, "Value"="Requires Hardware Tigger " ("hwtrigSel'd")) -> (error out=w419:errorcluster)  [unwired: 1 in, 1 out]
                      }
                    }
                  }
                  frame 1 {
                    n145 = call "sc5511a_list_soft_trigger.vi"("deviceHandle"=w424, "error in"=w423) -> ("deviceHandle"=w421:u32, "error out"=w422:errorcluster)  [unwired: 16 in]
                  }
                }
              }
            }
            n146 = call "Time Delay"("error in (no error)"=w388) -> ("error out"=w387:errorcluster)  [unwired: 10 in]
            n147 = property on="Trigger" class="Bool (strict)"(error in=w387, "Value"=FALSE ("Soft Tigger")) -> (error out=w384:errorcluster)  [unwired: 1 in, 1 out]
            n148 = call "sc5511a_get_device_status.vi"("deviceHandle"=w382, "error in"=w384) -> ("deviceHandle"=w383:u32, "Device Status"=w381:T11, "error out"=w385:errorcluster)  [unwired: 15 in]
          }
          event "Load Config", "Set As Default": Value Change {
            (unwired) u16 0 ("Direction")
            w435 = FALSE ("Soft Tigger")
            n149 = event-data() -> ()  [unwired: 1 in, 5 out]
            n150 = property on="List Mode Config" class="Clust (strict)"(error in=w461) -> (error out=w460:errorcluster, "Value"=w459:T4)  [unwired: 1 in, 1 out]
            n151 = call "sc5511a_list_mode_config.vi"("deviceHandle"=w462, "List Mode Config"=w459, "error in"=w460) -> ("deviceHandle"=w455:u32, "error out"=w458:errorcluster)  [unwired: 15 in]
            n152 = property on="Sweep Freq Parameter" class="Clust (strict)"(error in=w458) -> (error out=w452:errorcluster, "Value"=w457:T3)  [unwired: 1 in, 1 out]
            n153 = Unbundle(w457) -> ("Start Frequency"=w456:u64, "Stop Frequency"=w449:u64, "Step Frequency"=w448:u64)
            n154 = call "sc5511a_list_start_freq.vi"("deviceHandle"=w455, "List Start frequency"=w456, "error in"=w452) -> ("deviceHandle"=w454:u32, "error out"=w451:errorcluster)  [unwired: 15 in]
            n155 = call "sc5511a_list_stop_freq.vi"("deviceHandle"=w454, "RF frequency"=w449, "error in"=w451) -> ("deviceHandle"=w453:u32, "error out"=w450:errorcluster)  [unwired: 15 in]
            n156 = call "sc5511a_list_step_freq.vi"("deviceHandle"=w453, "List Step Frequency"=w448, "error in"=w450) -> ("deviceHandle"=w442:u32, "error out"=w447:errorcluster)  [unwired: 15 in]
            n157 = property on="Sweep/List Cycles" class="DigNum (strict)"(error in=w447) -> (error out=w445:errorcluster, "Value"=w446:u32)  [unwired: 1 in, 1 out]
            n158 = call "sc5511a_list_cycle_count.vi"("deviceHandle"=w442, "List Cycles"=w446, "error in"=w445) -> ("deviceHandle"=w441:u32, "error out"=w444:errorcluster)  [unwired: 15 in]
            n159 = property on="Dwell Period (ms)" class="DigNum (strict)"(error in=w444) -> (error out=w443:errorcluster, "Value"=w440:dbl)  [unwired: 1 in, 1 out]
            n160 = Multiply(x=w440, y=2.0) -> (x*y=w429:dbl)
            n161 = To Unsigned Long Integer(number=w429) -> (unsigned 32bit integer=w428:u32)
            n162 = call "sc5511a_list_dwell_time.vi"("deviceHandle"=w441, "List Dwell Time"=w428, "error in"=w443) -> ("deviceHandle"=w425:u32, "error out"=w426:errorcluster)  [unwired: 15 in]
            n163 = property on="Set As Default" class="Bool (strict)"(error in=w426) -> (error out=w439:errorcluster, "Value"=w437:bool)  [unwired: 1 in, 1 out]
            n164 = case shown="True" w437 {
              tunnel: w439 -> [w464 w468]
              tunnel: [w464 w467] -> w431
              tunnel: w425 -> [w463 w466]
              tunnel: [w463 w465] -> w438
              frame False {
              }
              frame True {
                n165 = call "sc5511a_store_default_state.vi"("deviceHandle"=w466, "error in"=w468) -> ("deviceHandle"=w465:u32, "error out"=w467:errorcluster)  [unwired: 16 in]
              }
            }
            n166 = call "Time Delay3"("error in (no error)"=w431) -> ("error out"=w430:errorcluster)  [unwired: 10 in]
            n167 = property on="Load Config" class="Bool (strict)"(error in=w430, "Value"=w435) -> (error out=w432:errorcluster)  [unwired: 1 in, 1 out]
            n168 = property on="Set As Default" class="Bool (strict)"(error in=w432, "Value"=w435) -> (error out=w436:errorcluster)  [unwired: 1 in, 1 out]
          }
          event "Download to Buffer": Value Change {
            n169 = event-data() -> ()  [unwired: 1 in, 5 out]
            n170 = Unbundle By Name(w470) -> ("Operate Status.RF Mode"=w469:u8)
            n171 = case shown="0, Default" w469 {
              selector: w469 -> [w479 w515]
              tunnel: w478 -> [w490 w513]
              tunnel: w477 -> [w489 w514]
              tunnel: [w487 w514] -> w476
              tunnel: [w486 w512] -> w472
              tunnel: [w479 w515] -> _
              frame 0, Default {
                # "0xFFFFFFFFFF to end buffer write"
                # "0 to reset the buffer to starting address\nand enable buffer write"
                n172 = call "sc5511a_list_buffer_write.vi"("deviceHandle"=w489, "List Frequency"=u64 0 ("Frequency"), "error in"=w490) -> ("deviceHandle"=w482:u32, "error out"=w485:errorcluster)  [unwired: 15 in]
                n173 = property on="Frequency List (2048 max)" class="Arr (strict)"(error in=w485) -> (error out=w483:errorcluster, "Value"=w484:u64[])  [unwired: 1 in, 1 out]
                n174 = for {
                  tunnel: w484 -> [w496] mode=indexing
                  tunnel: w483 -> [w498]
                  tunnel: w482 -> [w497]
                  tunnel: [w495] -> w480
                  tunnel: [w494] -> w481
                  i -> [w492]
                  stop <- w493 stop-if-true
                  n175 = Greater?(x=w492, y=2048) -> (0:w493:bool)
                  n176 = case shown="False" w493 {
                    tunnel: w498 -> [w507 w509]
                    tunnel: [w502 w509] -> w494
                    tunnel: w497 -> [w506 w508]
                    tunnel: w496 -> [w505 _]
                    tunnel: [w504 w508] -> w495
                    tunnel: w492 -> [w501 _]
                    frame False {
                      n177 = call "sc5511a_list_buffer_write.vi"("deviceHandle"=w506, "List Frequency"=w505, "error in"=w507) -> ("deviceHandle"=w504:u32, "error out"=w503:errorcluster)  [unwired: 15 in]
                      n178 = Increment(x=w501) -> (x+1=w500:i32)
                      n179 = property on="List Points" class="DigNum (strict)"(error in=w503, "Value"=w500) -> (error out=w502:errorcluster)  [unwired: 1 in, 1 out]
                    }
                    frame True {
                    }
                  }
                }
                n180 = call "sc5511a_list_buffer_write.vi"("deviceHandle"=w480, "List Frequency"=u64 1099511627775 ("Frequency"), "error in"=w481) -> ("deviceHandle"=w487:u32, "error out"=w486:errorcluster)  [unwired: 15 in]
              }
              frame 1 {
                n181 = property on="message 2" class="Str"(error in=w513, "Value"="List/Sweep On" ("message 2"), "Visible"=TRUE) -> (error out=w512:errorcluster)  [unwired: 1 in, 1 out]
              }
            }
            n182 = call "Time Delay2"("error in (no error)"=w472) -> ("error out"=w471:errorcluster)  [unwired: 10 in]
            n183 = property on="Download to Buffer" class="Bool (strict)"(error in=w471, "Value"=FALSE ("Download to Buffer")) -> (error out=w475:errorcluster)  [unwired: 1 in, 1 out]
          }
          event "Save Buffer to EEPROM", "Read EEPROM to Buffer": Value Change {
            w521 = FALSE ("Copy EEPROM to Buffer")
            n184 = event-data() -> ()  [unwired: 1 in, 5 out]
            n185 = Unbundle By Name(w517) -> ("Operate Status.RF Mode"=w516:u8)
            n186 = case shown="0, Default" w516 {
              tunnel: w525 -> [w531 w575]
              tunnel: w524 -> [w530 w577]
              tunnel: [w527 w576] -> w523
              tunnel: [w526 w577] -> w519
              frame 0, Default {
                n187 = property on="Read EEPROM to Buffer" class="Bool (strict)"(error in=w531) -> (error out=w528:errorcluster, "Value"=w529:bool)  [unwired: 1 in, 1 out]
                n188 = case shown="True" w529 {
                  tunnel: w530 -> [w545 w571]
                  tunnel: w528 -> [w539 w570]
                  tunnel: [w541 w569] -> w527
                  tunnel: [w543 w568] -> w526
                  frame True {
                    w546 = u16 1 items=["Buffer to EEPROM", "EEPROM to Buffer"] ("List Eeprom Config")
                    n189 = property on="List Points" class="DigNum (strict)"(error in=w539) -> (error out=w538:errorcluster, "Value"=w537:u32)  [unwired: 1 in, 1 out]
                    n190 = call "sc5511a_list_buffer_transfer.vi"("deviceHandle"=w545, "transfer mode"=w546, "error in"=w538) -> ("deviceHandle"=w542:u32, "error out"=w544:errorcluster)  [unwired: 15 in]
                    n191 = Greater Than 0?(x=w537) -> (x > 0?=w536:bool)
                    n192 = case shown="True" w536 {
                      tunnel: w544 -> [w549 w559]
                      tunnel: [w551 w558] -> w543
                      tunnel: w542 -> [w551 w557]
                      tunnel: [w549 w556] -> w540
                      tunnel: [u64[] [] w555] -> w535
                      tunnel: w537 -> [_ w554]
                      tunnel: [0 w553] -> w532
                      tunnel: [0 ("length") 1 ("length")] -> w534
                      frame False {
                      }
                      frame True {
                        n193 = while {
                          tunnel: w559 -> [w567]
                          tunnel: [w566] -> w556
                          tunnel: [w565] -> w558
                          tunnel: w557 -> [w564]
                          tunnel: [w563] -> w555 mode=indexing
                          tunnel: w554 -> [w562]
                          tunnel: [w560] -> w553
                          i -> [w560]
                          stop <- w561 continue-if-true
                          n194 = Less?(x=w560, y=w562) -> (x < y?=w561:bool)
                          n195 = call "sc5511a_list_buffer_read.vi"("deviceHandle"=w564, "address"=w560, "error in"=w567) -> ("deviceHandle"=w565:u32, "frequency"=w563:u64, "error out"=w566:errorcluster)  [unwired: 14 in]
                        }
                      }
                    }
                    n196 = Delete From Array(array=w535, length=w534, index=w532) -> (array with subset deleted=w533:u64[])  [unwired: 1 out]
                    n197 = property on="List Points" class="DigNum (strict)"("Value"=w532) -> ()  [unwired: 2 in, 2 out]
                    n198 = property on="Frequency List (2048 max)" class="Arr (strict)"(error in=w540, "Value"=w533) -> (error out=w541:errorcluster)  [unwired: 1 in, 1 out]
                  }
                  frame False {
                    w572 = u16 0 items=["Buffer to EEPROM", "EEPROM to Buffer"] ("List Eeprom Config")
                    n199 = call "sc5511a_list_buffer_transfer.vi"("deviceHandle"=w571, "transfer mode"=w572, "error in"=w570) -> ("deviceHandle"=w568:u32, "error out"=w569:errorcluster)  [unwired: 15 in]
                  }
                }
              }
              frame 1 {
                n200 = property on="message 2" class="Str"(error in=w575, "Value"="List Mode On" ("message 2"), "Visible"=TRUE) -> (error out=w576:errorcluster)  [unwired: 1 in, 1 out]
              }
            }
            n201 = property on="Read EEPROM to Buffer" class="Bool (strict)"(error in=w523, "Value"=w521) -> (error out=w522:errorcluster)  [unwired: 1 in, 1 out]
            n202 = property on="Save Buffer to EEPROM" class="Bool (strict)"(error in=w522, "Value"=w521) -> (error out=w520:errorcluster)  [unwired: 1 in, 1 out]
          }
        }
        n203 = Greater?(x=w175, y=u32 1500) -> (0:w173:bool)
        n204 = Multiply(x=w171, y=u16 1000) -> (x*y=w169:u16)
        n205 = Greater?(x=w170, y=w169) -> (0:w125:bool)
        n206 = local read "GetStatus"() -> (w167:bool)
        n207 = And(x=w167, y=w125) -> (x .and. y?=w123:bool)
        n208 = Unbundle By Name(w126) -> ("Operate Status.ListRuning"=w121:u8)
        n209 = case shown="True" w123 {
          tunnel: w178 -> [w201 w206]
          tunnel: w177 -> [w200 w205]
          tunnel: [w200 w203] -> w128
          tunnel: [w201 w204] -> w130
          tunnel: [w199 w202] -> w137
          tunnel: w126 -> [w199 _]
          frame False {
          }
          frame True {
            n210 = call "sc5511a_get_device_status.vi"("deviceHandle"=w206, "error in"=w205) -> ("deviceHandle"=w204:u32, "Device Status"=w202:T11, "error out"=w203:errorcluster)  [unwired: 15 in]
          }
        }
        n211 = Equal To 0?(x=w121) -> (x = 0?=w122:bool)
        n212 = And(x=w122, y=w125) -> (x .and. y?=w124:bool)
        n213 = Unbundle By Name(w137) -> ("Operate Status.Lock Mode"=w151:u8, "Operate Status.RFOutState"=w141:u8, "Operate Status.AutoPwrLevel"=w142:u8, "Operate Status.AlcMode"=w143:u8, "Operate Status.RF1 Standby"=w144:u8, "Operate Status.RF Mode"=w145:u8, "Operate Status.ListRuning"=w134:u8, "Operate Status.RF2 Standby"=w146:u8, "Operate Status.Ref Lock Enable"=w147:u8, "Operate Status.ExtRefDetected"=w148:u8, "Operate Status.RefOutSelect"=w149:u8, "PLL Status.Sum PLL"=w150:u8, "PLL Status.Crs assist PLL"=w155:u8, "PLL Status.Crs PLL"=w156:u8, "PLL Status.Crs Ref PLL"=w154:u8, "PLL Status.Fine PLL"=w158:u8, "Operate Status.Device Accessed"=w159:u8, "Operate Status.OverTempStatus"=w160:u8)
        n214 = case shown="True" w124 {
          tunnel: [w183 w190] -> w132
          tunnel: w133 -> [w183 _]
          tunnel: w131 -> [_ w190]
          tunnel: w130 -> [w182 w189]
          tunnel: [w182 w188] -> w129
          tunnel: w128 -> [w181 w187]
          tunnel: [w181 w185] -> w127
          frame False {
          }
          frame True {
            n215 = call "sc5511a_get_temperature.vi"("deviceHandle"=w189, "error in"=w187) -> ("deviceHandle"=w188:u32, "temperature"=w184:sgl, "error out"=w186:errorcluster)  [unwired: 15 in]
            n216 = property on="Temperature" class="DigNum (strict)"(error in=w186, "Value"=w184) -> (error out=w185:errorcluster)  [unwired: 1 in, 1 out]
          }
        }
        n217 = case shown="True" w173 {
          selector: w173 -> [_ w195]
          tunnel: w127 -> [w192 w198]
          tunnel: [w192 w197] -> w162
          tunnel: w165 -> [w191 _]
          tunnel: [w191 w193] -> w166
          tunnel: w131 -> [_ w193]
          frame False {
          }
          frame True {
            n218 = Not(x=w195) -> (.not. x?=w194:bool)
            n219 = property on="message" class="Str"(error in=w198, "Visible"=w194) -> (error out=w196:errorcluster)  [unwired: 1 in, 1 out]
            n220 = property on="message 2" class="Str"(error in=w196, "Visible"=w194) -> (error out=w197:errorcluster)  [unwired: 1 in, 1 out]
          }
        }
        n221 = Not Equal To 0?(x=w151) -> (x != 0?=w152:bool)
        n222 = Select(t=w155, s=w152, f=w156) -> (s? t:f=w153:u8)
        n223 = And(x=w153, y=w154) -> (x .and. y?=w157:u8)
        n224 = Not Equal To 0?(x=w150) -> (x != 0?=w138:bool)
        n225 = Not Equal To 0?(x=w157) -> (x != 0?=w139:bool)
        n226 = Not Equal To 0?(x=w158) -> (x != 0?=w140:bool)
        n227 = Unbundle By Name(w162) -> ("status"=w163:bool)
        n228 = Bundle By Name(cluster=T9 {"Synth Mode"=0, "RF Out"=0, "Auto Power"=0, "ALC Mode"=0, "Standby"=0, "Rf RF Mode"=0, "List Mode State"=0, "RF2 Standby"=0, "Ref Lock Enable"=0, "Ext Ref Detected"=0, "Ref out mode"=0, "Main PLL"=1, "Crs PLL"=1, "Fine PLL"=1, "device accessed"=0, "Over Temp"=0, "MainLED"=FALSE, "CrsLED"=FALSE, "FineLED"=FALSE} ("Device Status"), "Synth Mode"=w151, "RF Out"=w141, "Auto Power"=w142, "ALC Mode"=w143, "Standby"=w144, "Rf RF Mode"=w145, "List Mode State"=w134, "RF2 Standby"=w146, "Ref Lock Enable"=w147, "Ext Ref Detected"=w148, "Ref out mode"=w149, "Main PLL"=w150, "Crs PLL"=w157, "Fine PLL"=w158, "device accessed"=w159, "Over Temp"=w160, "MainLED"=w138, "CrsLED"=w139, "FineLED"=w140) -> (w136:T9)
        n229 = Or(x=w163, y=w164) -> (x .or. y?=w161:bool)
        n230 = property on="Device Status" class="Clust (strict)"("Value"=w136) -> ()  [unwired: 2 in, 2 out]
      }
      n231 = call "sc5511a_close_device.vi"("deviceHandle"=w97, "error in (no error)"=w98) -> ("error out"=w96:errorcluster)  [unwired: 17 in]
    }
    frame Error {
    }
  }
  n232 = Unbundle By Name(w7) -> ("status"=w3:bool)
  n233 = case shown="True" w3 {
    selector: w3 -> [_ w579]
    frame False {
    }
    frame True {
      n234 = property on="error out" class="Clust (strict)"("Visible"=w579) -> ()  [unwired: 2 in, 2 out]
      n235 = property on="Tab Control" class="TabCtl (strict)"("Value"=T1."Device Info" ("Tab Control")) -> ()  [unwired: 2 in, 2 out]
    }
  }
  n236 = property on="On" class="Bool (strict)"(error in=w7, "Value"=FALSE ("Visible")) -> (error out=→"error out":errorcluster)  [unwired: 1 in, 1 out]
